vi "Logging Flatten.vi"(1 "In":T1) -> (0 "Out":T4)   [LabVIEW 2012, in "femtoRoboLib.lvlib"]
uses:
  Log Entry - Converted.ctl
  Log Entry.ctl
  Log Value Type.ctl
  Log Value Cluster.ctl
  femtoRoboLib.lvlib
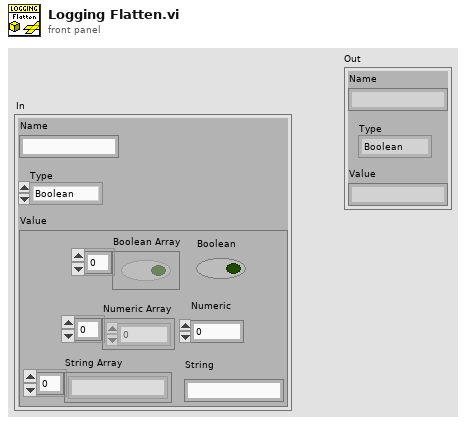
[diagram p1: front panel]
types:
  T1 = typedef "femtoRoboLib.lvlib/Log Entry.ctl" = cluster{"Name":string, "Type":T2, "Value":T3}
  T2 = typedef "femtoRoboLib.lvlib/Log Value Type.ctl" = enum16{"Boolean", "Numeric", "String", "Boolean Array", "Numeric Array", "String Array"}
  T3 = typedef "femtoRoboLib.lvlib/Log Value Cluster.ctl" = cluster{"Boolean Array":bool[], "Boolean":bool, "Numeric Array":dbl[], "Numeric":dbl, "String Array":string[], "String":string}
  T4 = typedef "femtoRoboLib.lvlib/Log Entry - Converted.ctl" = cluster{"Name":string, "Type":enum16{"Boolean", "Numeric", "String", "Boolean Array", "Numeric Array", "String Array"}, "Value":string}
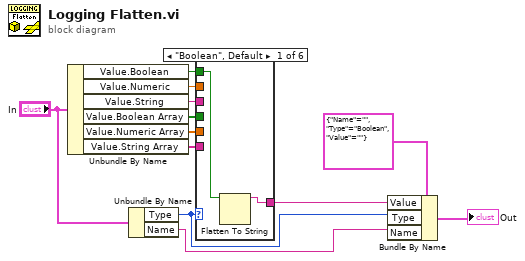
[diagram p0: block diagram]
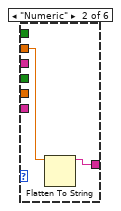
[diagram p2: hidden frame]
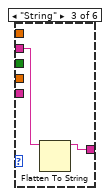
[diagram p3: hidden frame]
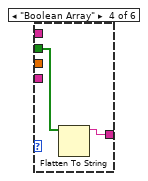
[diagram p4: hidden frame]
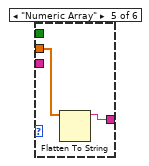
[diagram p5: hidden frame]
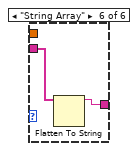
[diagram p6: hidden frame]
diagram:
  n1 = Unbundle By Name("In") -> ("Value.Boolean"=w12:bool, "Value.Numeric"=w11:dbl, "Value.String"=w10:string, "Value.Boolean Array"=w9:bool[], "Value.Numeric Array"=w8:dbl[], "Value.String Array"=w7:string[])
  n2 = Unbundle By Name("In") -> ("Type"=w4:T2, "Name"=w6:string)
  n3 = case shown="\"Boolean\", Default" w4 {
    tunnel: w12 -> [w13 _ _ _ _ _]
    tunnel: w11 -> [_ w16 _ _ _ _]
    tunnel: w10 -> [_ _ w18 _ _ _]
    tunnel: w9 -> [_ _ _ w20 _ _]
    tunnel: w8 -> [_ _ _ _ w21 _]
    tunnel: w7 -> [_ _ _ _ _ w23]
    tunnel: [w14 w15 w17 w19 w22 w24] -> w3
    frame "Boolean", Default {
      n4 = Flatten To String(anything=w13) -> (data string=w14:string)  [unwired: 3 in, 2 out]
    }
    frame "Numeric" {
      n5 = Flatten To String(anything=w16) -> (data string=w15:string)  [unwired: 3 in, 2 out]
    }
    frame "String" {
      n6 = Flatten To String(anything=w18) -> (data string=w17:string)  [unwired: 3 in, 2 out]
    }
    frame "Boolean Array" {
      n7 = Flatten To String(anything=w20) -> (data string=w19:string)  [unwired: 3 in, 2 out]
    }
    frame "Numeric Array" {
      n8 = Flatten To String(anything=w21) -> (data string=w22:string)  [unwired: 3 in, 2 out]
    }
    frame "String Array" {
      n9 = Flatten To String(anything=w23) -> (data string=w24:string)  [unwired: 3 in, 2 out]
    }
  }
  n10 = Bundle By Name(cluster=T4 {"Name"="", "Type"=enum."Boolean", "Value"=""} ("Out"), "Value"=w3, "Type"=w4, "Name"=w6) -> (→"Out":T4)
